vi "get all scores.vi"() -> ()   [LabVIEW 2022 SP3]
uses:
  FullHighscoreIndicator.ctl
  HighscoreIndicator.ctl
  FullHighScoreScoreIndicator.ctl
  HighscoreIndicatorYes.ctl
panel:
  out "High Score Scores":T1 caption="HIGH SCORE"
  out "High Score Names":T3 caption="HIGH SCORE"
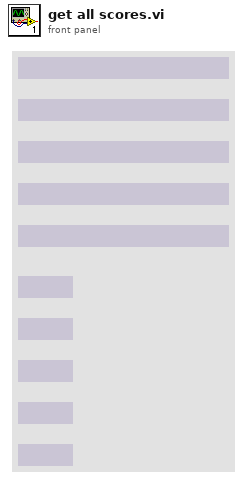
[diagram p1: front panel]
types:
  T1 = typedef "FullHighScoreScoreIndicator.ctl" = T2[]
  T2 = typedef "HighscoreIndicatorYes.ctl" = string
  T3 = typedef "FullHighscoreIndicator.ctl" = T4[]
  T4 = typedef "HighscoreIndicator.ctl" = string
  T5 = enum16{"open", "open or create", "create or replace", "create", "open (read-only)"}
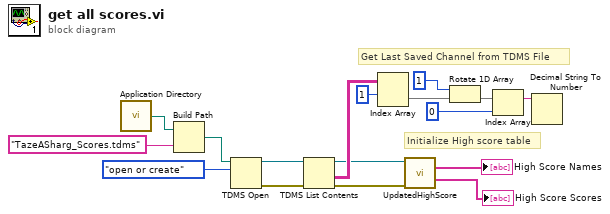
[diagram p0: block diagram]
diagram:
  # "Get Last Saved Channel from TDMS File"
  # "Initialize High score table"
  n1 = call <vilib>:"Application Directory.vi"() -> ("Application Directory"=w17:path)
  n2 = Build Path(base path=w17, name or relative path="TazeASharg_Scores.tdms") -> (appended path=w16:path)
  n3 = TDMS Open(10:T5."open or create" ("operation (0:open)"), 11:w16) -> (0:w13:errorcluster, 3:w14:refnum<k34>)  [unwired: 5 in]
  n4 = TDMS List Contents(4:w13, 7:w14) -> (0:w4:errorcluster, 1:w7:string[][], 3:w5:refnum<k34>)  [unwired: 1 in, 1 out]
  n5 = Index Array(array=w7, index (row)=1) -> (element=w12:string[])  [unwired: 1 in]
  n6 = call "UpdatedHighScore.vi"("tdms file"=w5, "error in (no error)"=w4) -> ("Names"=→"High Score Names":string[], "Scores"=→"High Score Scores":string[])  [unwired: 10 in, 2 out]
  n7 = Rotate 1D Array(1:w12, 2:1 ("n")) -> (0:w10:string[])
  n8 = Index Array(array=w10, index=0) -> (element=w6:string)
  n9 = Decimal String To Number(string=w6) -> ()  [unwired: 2 in, 2 out]
